vi "Run Tests using Transcriptor.vi"() -> ()   [LabVIEW 2014]
panel:
  in  "error in":errorcluster
  out "error out":errorcluster
  out "transcripted code":string
  in  "vi path":path=path "C:/Users/lubo/Documents/LabView/LabVIEW-Universal-Transcriptor-ServoLibrary/Debug Test/Test attach 1.vi"
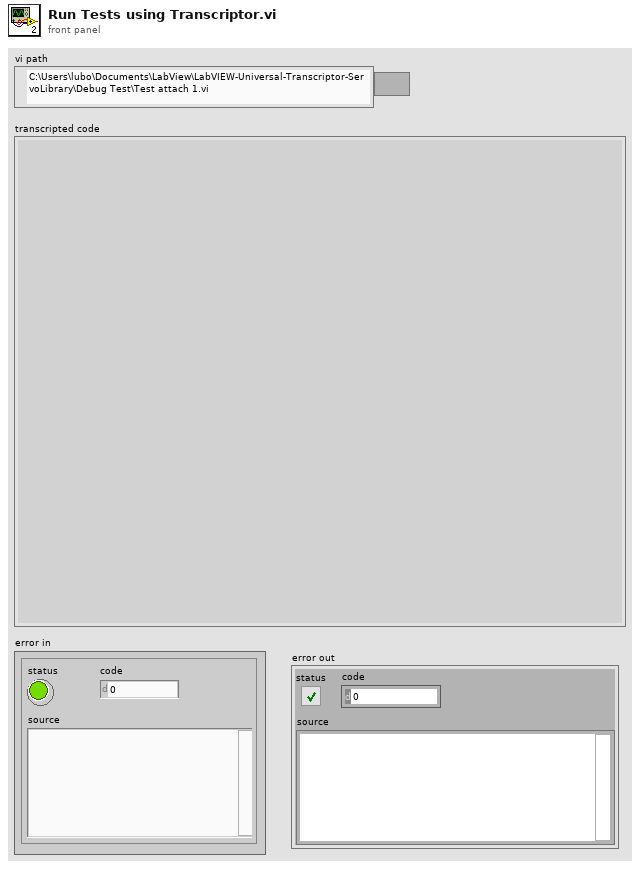
[diagram p1: front panel]
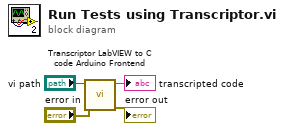
[diagram p0: block diagram]
diagram:
  n1 = call <vilib>:"Transcriptor LabVIEW to C code Arduino Frontend.vi"("error in"="error in", "vi path"="vi path") -> ("error out"=→"error out":errorcluster, "transcripted code"=→"transcripted code":string)  [unwired: 8 in]
